vi "Set Tag on Selected Object.vi"() -> ()   [LabVIEW 2012]
doc: "Finds a selected object and allows the user to tag it."
uses:
  Scripting Tools.lvlib
panel:
  in  "error IO":errorcluster
  out "Object Tagged ?":bool
  in  "Cancel":bool
  in  "Apply No Close":bool
  in  "Apply and Close":bool
  in  "Tag Value":string
  in  "Tag Name":string(combo)
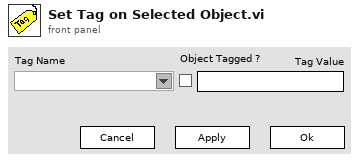
[diagram p1: front panel]
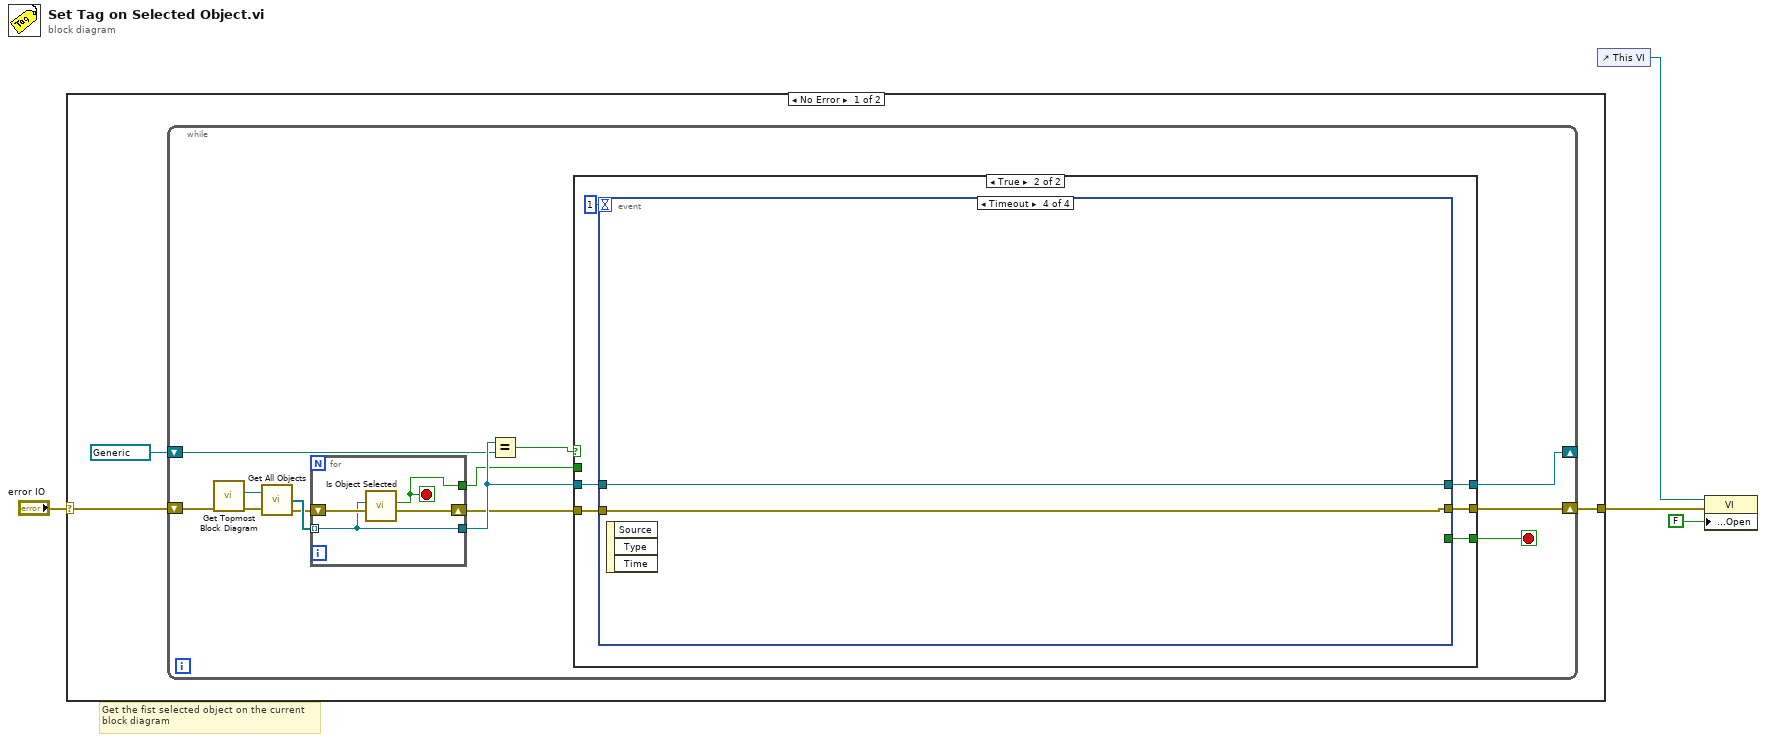
[diagram p0: block diagram]
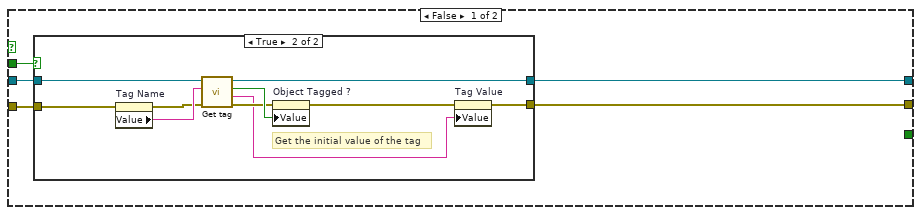
[diagram p2: hidden frame]
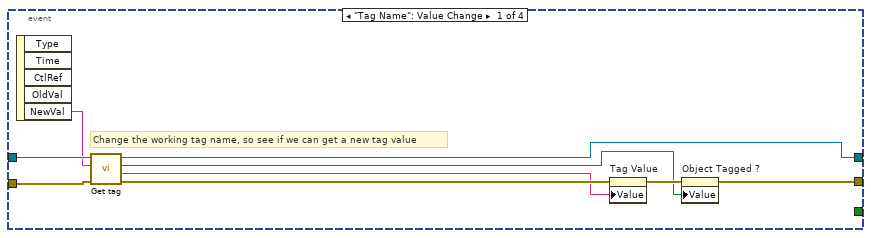
[diagram p4: hidden frame]
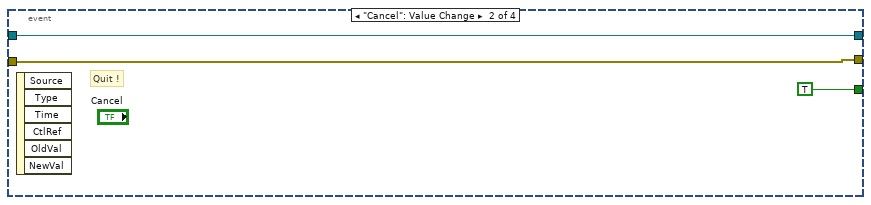
[diagram p5: hidden frame]
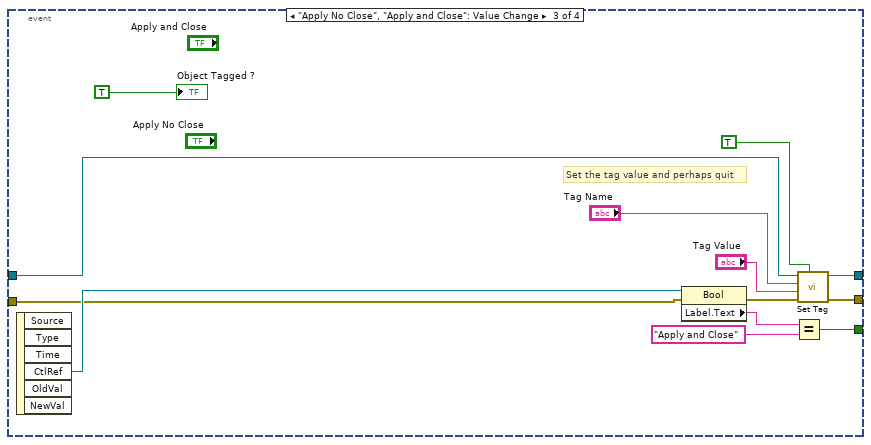
[diagram p6: hidden frame]
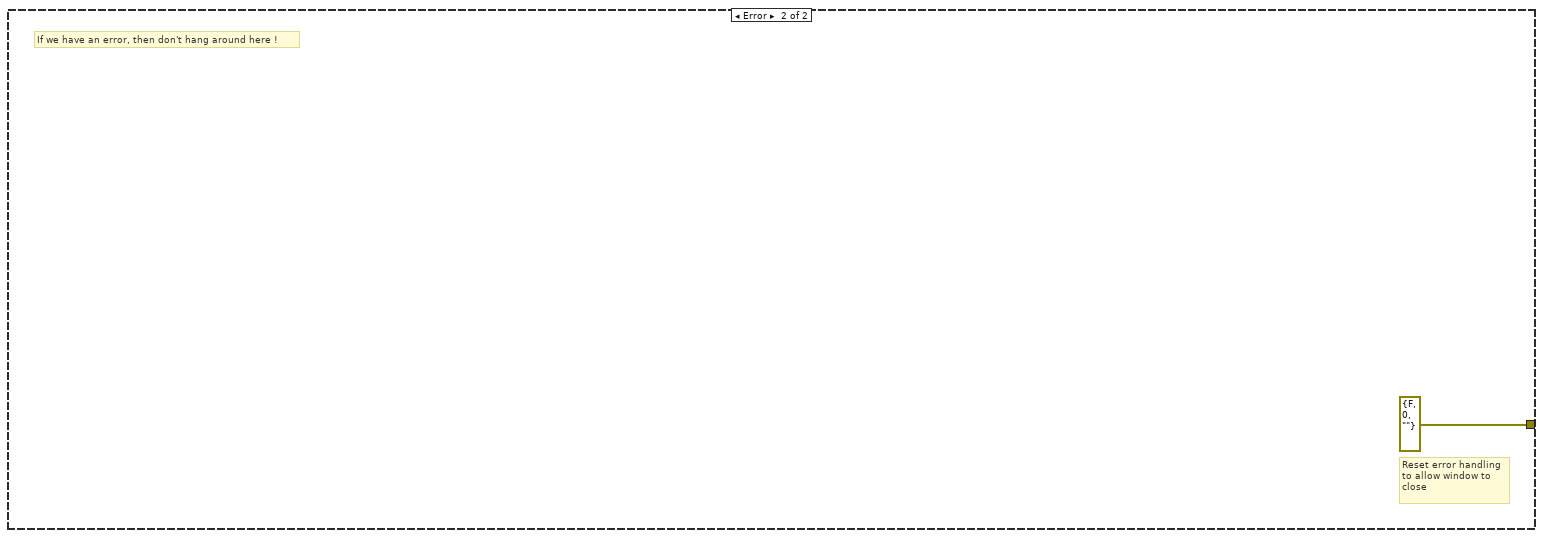
[diagram p7: hidden frame]
diagram:
  # "Get the fist selected object on the current\nblock diagram"
  n1 = case shown="No Error" "error IO" {
    selector: "error IO" -> [w7 _]
    tunnel: [w6 errorcluster {"status"=FALSE, "code"=0, "source"=""} ("error IO")] -> w4
    frame No Error {
      n2 = while {
        shift-right: [w20] -> w6
        shift-left: w7 -> [w10]
        shift-right: [w19] -> _
        shift-left: refnum<vi> refnum ("reference Out") -> [w12]
        stop <- w18 stop-if-true
        n3 = call "Get Topmost Block Diagram.vi"("error in (no error)"=w10) -> ("error out"=w14:errorcluster, "Reference to Diagram"=w15:refnum<vi>)  [unwired: 9 out]
        n4 = call "Get All Objects.vi"("Diagram In"=w15, "error in"=w14) -> ("All Objects"=w17:refnum<vi>[], "error out"=w16:errorcluster)  [unwired: 1 out]
        n5 = for {
          shift-right: [w22] -> w9
          shift-left: w16 -> [w24]
          tunnel: w17 -> [w23] mode=indexing
          tunnel: [w23] -> w13
          tunnel: [w21] -> w11
          stop <- w21 stop-if-true
          n6 = call "Is Object Selected.vi"("error in (no error)"=w24, "GObject Reference"=w23) -> ("error out"=w22:errorcluster, "Selected"=w21:bool)  [unwired: 8 out]
        }
        n7 = Equal?(x=w13, y=w12) -> (x = y?=w8:bool)
        n8 = case shown="True" w8 {
          tunnel: w9 -> [w25 w47]
          tunnel: w13 -> [w28 w46]
          tunnel: [w26 w45] -> w20
          tunnel: [w27 w44] -> w19
          tunnel: [_ w43] -> w18
          tunnel: w11 -> [w29 _]
          frame False {
            n9 = case shown="True" w29 {
              tunnel: w28 -> [w30 w35]
              tunnel: [w30 w34] -> w27
              tunnel: [w31 w33] -> w26
              tunnel: w25 -> [w31 w32]
              frame False {
              }
              frame True {
                # "Get the initial value of the tag"
                n10 = property on="Tag Name" class="CmbBox"(error in=w32) -> (error out=w40:errorcluster, "Value"=w41:string)  [unwired: 1 in, 1 out]
                n11 = call "Get tag.vi"("error in (no error)"=w40, "TagName"=w41, "reference"=w35) -> ("error out"=w38:errorcluster, "Tag Value"=w36:string, "Tag Found ?"=w39:bool, "reference Out"=w34:refnum<vi>)  [unwired: 5 out]
                n12 = property on="Object Tagged ?" class="Bool (strict)"(error in=w38, "Value"=w39) -> (error out=w37:errorcluster)  [unwired: 1 in, 1 out]
                n13 = property on="Tag Value" class="Str"(error in=w37, "Value"=w36) -> (error out=w33:errorcluster)  [unwired: 1 in, 1 out]
              }
            }
          }
          frame True {
            n14 = event shown="[3] Timeout" {
              selector: _ -> [_ _ _ _]
              dyn-events: _ -> [_ _ _ _]
              timeout: 1 -> [_ _ _ _]
              tunnel: w47 -> [w56 w58 w62 w74]
              tunnel: w46 -> [w55 w59 w71 w73]
              tunnel: [w49 w58 w68 w74] -> w45
              tunnel: [w48 w59 w72 w73] -> w44
              tunnel: [_ TRUE w61 _] -> w43
              event "Tag Name": Value Change {
                # "Change the working tag name, so see if we can get a new tag value"
                n15 = event-data() -> ("NewVal"=w52:string)  [unwired: 5 out]
                n16 = call "Get tag.vi"("error in (no error)"=w56, "TagName"=w52, "reference"=w55) -> ("error out"=w54:errorcluster, "Tag Value"=w53:string, "Tag Found ?"=w50:bool, "reference Out"=w48:refnum<vi>)  [unwired: 5 out]
                n17 = property on="Tag Value" class="Str"(error in=w54, "Value"=w53) -> (error out=w51:errorcluster)  [unwired: 1 in, 1 out]
                n18 = property on="Object Tagged ?" class="Bool (strict)"(error in=w51, "Value"=w50) -> (error out=w49:errorcluster)  [unwired: 1 in, 1 out]
              }
              event "Cancel": Value Change {
                # "Quit !"
                n19 = event-data() -> ()  [unwired: 7 out]
              }
              event "Apply No Close", "Apply and Close": Value Change {
                # "Set the tag value and perhaps quit"
                n20 = event-data() -> ("CtlRef"=w65:refnum<vi>)  [unwired: 6 out]
                n21 = property class="Bool"(reference=w65, error in=w62) -> (error out=w60:errorcluster, "Label.Text"=w64:string)  [unwired: 1 out]
                n22 = Equal?(x=w64, y="Apply and Close") -> (x = y?=w61:bool)
                n23 = call "Set Tag.vi"("Persistant"=TRUE, "error in (no error)"=w60, "Tag Value"="Tag Value", "TagName"="Tag Name", "reference"=w71) -> ("error out"=w68:errorcluster, "reference Out"=w72:refnum<vi>)  [unwired: 5 out]
                "Object Tagged ?" <- TRUE ("Object Tagged ?")
              }
              event Timeout {
                n24 = event-data() -> ()  [unwired: 4 out]
              }
            }
          }
        }
      }
    }
    frame Error {
      # "Reset error handling\nto allow window to\nclose"
      # "If we have an error, then don't hang around here !"
    }
  }
  n25 = control-ref of="This VI"() -> (w3:refnum<vi>)
  n26 = property class="VI"(reference=w3, error in=w4, "Front Panel.Open"=FALSE ("Front Panel Window:Open")) -> ()  [unwired: 2 out]
